vi "Forward_Kinematics (geo and matrix).vi"(8 "geometry":cluster{"L 1":dbl, "L 2":dbl, "q":dbl[]}={"L 1"=30.0, "L 2"=35.0, "q"=[20.0, -40.0]}, 9 "geometry?":bool, 10 "arms":T2(array[cluster])=[{"Translation"={"X"=0.0, "Y"=0.0, "Z"=0.0}, "Axis"=enum."z", "Angle (degrees)"=20.0}, {"Translation"={"X"=30.0, "Y"=0.0, "Z"=0.0}, "Axis"=enum."z", "Angle (degrees)"=-40.0}, {"Translation"={"X"=35.0, "Y"=0.0, "Z"=0.0}, "Axis"=enum."z", "Angle (degrees)"=0.0}] {"Angle (degrees)" scale=0.0..180.0}, 11 "picture in":picture) -> (0 "end (2D)":cluster{"x":dbl, "y":dbl}, 1 "end effector":cluster{"X":dbl, "Y":dbl}={"X"=61.080020351084045, "Y"=-1.710100716628343}, 3 "2D Picture":picture)   [LabVIEW 2024]
uses:
  <vilib>/Analysis/Matrix/Datatypes/RealMatrix.ctl
  <vilib>/Analysis/baseanly.llb/Real A x B.vi
  <vilib>/Analysis/NI_AALBase.lvlib
  <vilib>/Analysis/Matrix/NI_Matrix.lvlib
panel:
  out "x1y1":cluster{"x1":dbl, "y1":dbl}
  out "xy":cluster{"x":dbl, "y":dbl}
  out "array w/ subset deleted":T1(array[cluster])
  out "appended array":cluster{"x":dbl, "y":dbl}[](array[cluster])
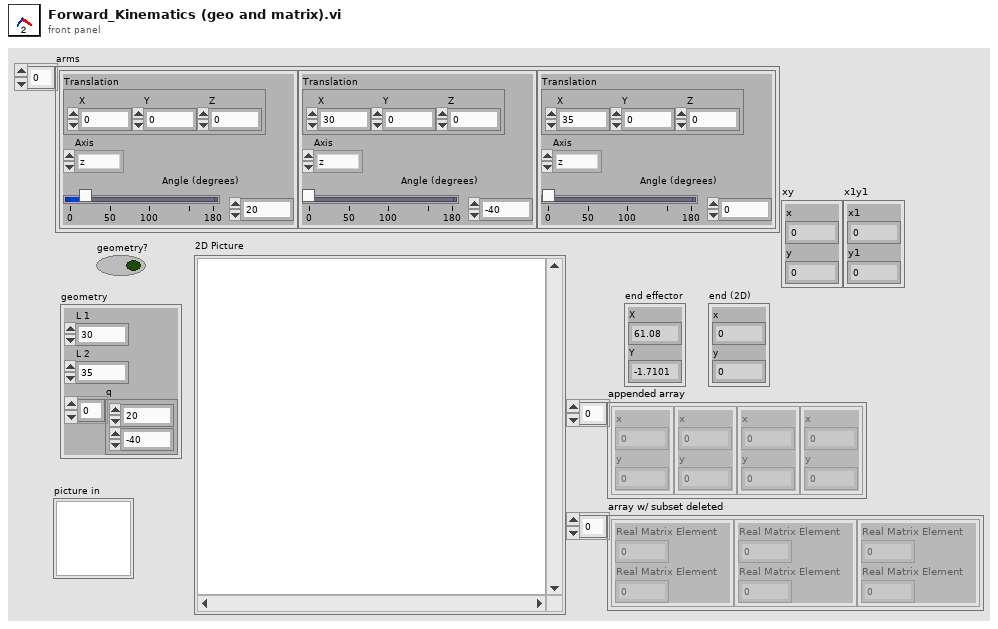
[diagram p1: front panel]
types:
  T1 = cluster{"Real Matrix Element":dbl, "Real Matrix Element":dbl}[]
  T2 = cluster{"Translation":cluster{"X":dbl, "Y":dbl, "Z":dbl}, "Axis":enum16{"x", "y", "z"}, "Angle (degrees)":dbl}[]
  T3 = typedef "NI_Matrix.lvlib/RealMatrix.ctl" = dbl[][]
  T4 = cluster{"Real Matrix Element":dbl, "Real Matrix Element":dbl}
  T5 = cluster{"Width":u16, "Style":enum32{"Solid", "Dash", "Dot", "DashDot", "DashDotDot"}}
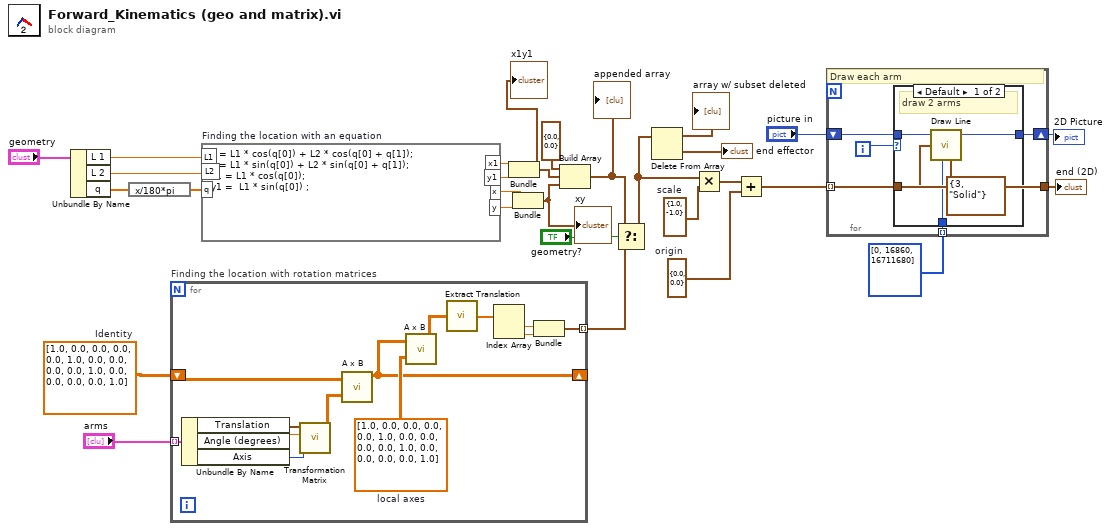
[diagram p0: block diagram]
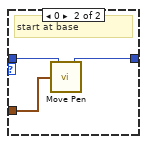
[diagram p2: hidden frame]
diagram:
  w9 = T3 [[1.0, 0.0, 0.0, 0.0], [0.0, 1.0, 0.0, 0.0], [0.0, 0.0, 1.0, 0.0], [0.0, 0.0, 0.0, 1.0]]  # Identity
  w14 = cluster{"x":dbl, "y":dbl} {"x"=1.0, "y"=-1.0}  # scale
  w13 = cluster{"x":dbl, "y":dbl} {"x"=0.0, "y"=0.0}  # origin
  n1 = Unbundle By Name("geometry") -> ("L 1"=w25:dbl, "L 2"=w26:dbl, "q"=w27:dbl[])
  n2 = expression code="x/180*pi"(w27) -> (w5:dbl[])
  n3 = for "Finding the location with rotation matrices" {
    tunnel: "arms" -> [w36] mode=indexing
    shift-right: [w34] -> _
    shift-left: w9 -> [w35]
    tunnel: [w29] -> w8 mode=indexing
    w37 = T3 [[1.0, 0.0, 0.0, 0.0], [0.0, 1.0, 0.0, 0.0], [0.0, 0.0, 1.0, 0.0], [0.0, 0.0, 0.0, 1.0]]  # local axes
    n4 = Unbundle By Name(w36) -> ("Translation"=w41:cluster{"X":dbl, "Y":dbl, "Z":dbl}, "Angle (degrees)"=w40:dbl, "Axis"=w39:enum16{"x", "y", "z"})
    n5 = call <userlib>:"Transformation Matrix.vi"("Axis"=w39, "Angle (degrees)"=w40, "Translation"=w41) -> ("Transformation Matrix"=w38:T3)  [unwired: 8 in]
    n6 = call-poly <vilib>:"A x B.vi"("B"=w38, "A"=w35) -> ("A x B"=w34:T3)  [unwired: 1 out]
    n7 = call-poly <vilib>:"A x B.vi"("B"=w37, "A"=w34) -> ("A x B"=w33:T3)  [unwired: 1 out]
    n8 = call <userlib>:"Extract Translation.vi"("Transformation matrix"=w33) -> ("translation"=w32:dbl[])
    n9 = Index Array(array=w32) -> (element #1=w31:dbl, element #2=w30:dbl)  [unwired: 2 in]
    n10 = Bundle("Real Matrix Element"=w31, "Real Matrix Element"=w30) -> (w29:T4)  [unwired: 1 in]
  }
  n11 = formula code="x = L1 * cos(q[0]) + L2 * cos(q[0] + q[1]);\ny = L1 * sin(q[0]) + L2 * sin(q[0] + q[1]);\nx1 = L1 * cos(q[0]);\ny1 =  L1 * sin(q[0]) ;" "Finding the location with an equation"("q"=w5, "L1"=w25, "L2"=w26) -> ("x"=w24:dbl, "y"=w23:dbl, "x1"=w22:dbl, "y1"=w21:dbl)
  n12 = Bundle("x1"=w22, "y1"=w21) -> (w20:cluster{"x1":dbl, "y1":dbl})  [unwired: 1 in]
  "x1y1" <- w20
  n13 = Bundle("x"=w24, "y"=w23) -> (w19:cluster{"x":dbl, "y":dbl})  [unwired: 1 in]
  "xy" <- w19
  n14 = Build Array(cluster{"x":dbl, "y":dbl} {"x"=0.0, "y"=0.0} ("y"), w20, w19) -> (w7:cluster{"x":dbl, "y":dbl}[])
  "appended array" <- w7
  n15 = Select(t=w7, s="geometry?", f=w8) -> (s? t:f=w4:T1)
  n16 = Delete From Array(array=w4) -> (deleted portion=→"end effector":T4, array with subset deleted=→"array w/ subset deleted":T1)  [unwired: 2 in]
  n17 = Multiply(x=w4, y=w14) -> (x*y=w12:cluster{dbl, dbl}[])
  n18 = Add(x=w12, y=w13) -> (x+y=w11:cluster{dbl, dbl}[])
  n19 = for {
    shift-right: [w44] -> w17
    shift-left: "picture in" -> [w45]
    tunnel: u32[] [0, 16860, 16711680] -> [w43] mode=indexing
    tunnel: w11 -> [w42] mode=indexing
    tunnel: [w42] -> w2
    i -> [w46]
    # "Draw each arm"
    n20 = case shown="Default" w46 {
      tunnel: w45 -> [w51 w54]
      tunnel: [w50 w53] -> w44
      tunnel: w42 -> [w49 w52]
      tunnel: w43 -> [w48 _]
      frame Default {
        # "draw 2 arms"
        n21 = call <vilib>:"Draw Line.vi"("picture"=w51, "end point"=w49, "color(black)"=w48, "pen"=T5 {"Width"=3, "Style"=enum."Solid"}) -> ("new picture"=w50:picture)  [unwired: 5 in]
      }
      frame 0 {
        # "start at base"
        n22 = call <vilib>:"Move Pen.vi"("new position"=w52, "picture"=w54) -> ("new picture"=w53:picture)  [unwired: 3 in]
      }
    }
  }
  "2D Picture" <- w17
  "end (2D)" <- w2
